vi "UHR-Fleezers Control (host) - 10.4.vi"() -> ()   [LabVIEW 2011] (continued)
            n1300 = local write "Manipulating Trap"(TRUE ("Manipulating Trap")) -> ()
            n1301 = local write "Coords"(T7 {"Horizontal"=0, "Vertical"=0} ("Coords")) -> ()
            n1302 = while {
              tunnel: w1981 -> [w1986]
              tunnel: w1979 -> [w1985]
              tunnel: w1977 -> [w1984]
              tunnel: w1976 -> [w1983]
              tunnel: w1975 -> [w1982]
              stop <- w1987 stop-if-true
              n1303 = event shown="[0] \"Pane\": Mouse Move" {
                selector: _ -> [_ _]
                dyn-events: _ -> [_ _]
                timeout: _ -> [_ _]
                tunnel: ["Force Manip Abort" w2051] -> w1987
                tunnel: w1986 -> [w1994 _]
                tunnel: w1985 -> [w1992 _]
                tunnel: w1984 -> [w1991 _]
                tunnel: w1983 -> [w1990 _]
                tunnel: w1982 -> [w1989 _]
                event Mouse Move {
                  n1304 = event-data() -> ("Time"=w1995:u32, "Coords"=w1996:T7)  [unwired: 3 out]
                  n1305 = Less?(x=w1995, y=w1994) -> (x < y?=w1993:bool)
                  n1306 = case "Makes sure old motion events prior to mouse click aren't used" shown="False" w1993 {
                    tunnel: w1996 -> [w2038 _]
                    tunnel: w1992 -> [w2039 _]
                    tunnel: w1991 -> [w2016 _]
                    tunnel: w1990 -> [w2012 _]
                    tunnel: w1989 -> [w2011 _]
                    frame False {
                      n1307 = Subtract(x=w2038, y=w2039) -> (x-y=w2037:T7)
                      "Coords" <- w2037
                      n1308 = local read "Y RF Frequency Limits (MHz)"() -> (w1997:T16)
                      n1309 = To Double Precision Float(number=w2037) -> (double precision float=w2036:cluster{"Horizontal":dbl, "Vertical":dbl})
                      n1310 = Multiply(x=cluster{"Horizontal":dbl, "Vertical":dbl} {"Horizontal"=-1.0, "Vertical"=1.0}, y="Manipulation Scaling") -> (x*y=w2032:cluster{"Horizontal":dbl, "Vertical":dbl})
                      n1311 = local read "X RF Frequency Limits (MHz)"() -> (w1998:T16)
                      n1312 = Multiply(x=w2036, y=w2032) -> (x*y=w2034:cluster{"Horizontal":dbl, "Vertical":dbl})
                      n1313 = Unbundle By Name(w2034) -> ("Horizontal"=w2029:dbl, "Vertical"=w2033:dbl)
                      n1314 = Unbundle By Name(w1997) -> ("Maximum"=w2000:dbl, "Minimum"=w1999:dbl)
                      n1315 = Boolean To (0,1)(Boolean="Manip. X?") -> (0, 1=w2027:i16)
                      n1316 = Boolean To (0,1)(Boolean="Manip. Y?") -> (0, 1=w2024:i16)
                      n1317 = local read "BD 1 Frequency 2 (MHz)"() -> (w2014:dbl)
                      n1318 = Multiply(x=w2033, y=w2024) -> (x*y=w2026:dbl)
                      n1319 = Multiply(x=w2027, y=w2029) -> (x*y=w2030:dbl)
                      n1320 = local read "BD 2 Frequency 2 (MHz)"() -> (w2013:dbl)
                      n1321 = Unbundle By Name(w1998) -> ("Maximum"=w2002:dbl, "Minimum"=w2001:dbl)
                      n1322 = Add(x=w2011, y=w2026) -> (x+y=w2004:dbl)
                      n1323 = Add(x=w2012, y=w2030) -> (x+y=w2006:dbl)
                      n1324 = In Range and Coerce(upper limit=w2002, x=w2006, lower limit=w2001) -> (coerced(x)=w2005:dbl)  [unwired: 1 out]
                      n1325 = In Range and Coerce(upper limit=w2000, x=w2004, lower limit=w1999) -> (coerced(x)=w2003:dbl)  [unwired: 1 out]
                      n1326 = Subtract(x=w2005, y=w2014) -> (x-y=w2023:dbl)
                      n1327 = Subtract(x=w2003, y=w2013) -> (x-y=w2022:dbl)
                      n1328 = Square(x=w2023) -> (x^2=w2021:dbl)
                      n1329 = Square(x=w2022) -> (x^2=w2020:dbl)
                      n1330 = Add(x=w2021, y=w2020) -> (x+y=w2019:dbl)
                      n1331 = Square Root(x=w2019) -> (sqrt(x)=w2015:dbl)
                      n1332 = In Range and Coerce(upper limit="Limit Max (MHz)", x=w2015, lower limit="Limit Min (MHz)") -> (In Range?=w2008:bool)  [unwired: 1 out]
                      n1333 = Not(x="Limits Enable") -> (.not. x?=w2007:bool)
                      n1334 = Or(x=w2008, y=w2007) -> (x .or. y?=w2009:bool)
                      n1335 = case shown="True" w2009 {
                        tunnel: w2016 -> [_ w2049]
                        tunnel: w2015 -> [_ w2040]
                        tunnel: w2005 -> [_ w2047]
                        tunnel: w2014 -> [_ w2046]
                        tunnel: w2003 -> [_ w2045]
                        tunnel: w2013 -> [_ w2044]
                        tunnel: w1998 -> [_ w2042]
                        tunnel: w1997 -> [_ w2041]
                        frame False {
                        }
                        frame True {
                          n1336 = local read "BD 1 Frequency 3 (MHz)"() -> (w2048:dbl)
                          n1337 = local read "BD 2 Frequency 3 (MHz)"() -> (w2043:dbl)
                          n1338 = local write "Trap Delta (MHz)"(w2040) -> ()
                          n1339 = call "set RF board frequency - interlace.vi"("Board 2 Frequency Limits"=w2041, "Board 1 Frequency Limits"=w2042, "FPGA VI Reference In"=w2049, "Board 2 Frequency 3 (MHz)"=w2043, "Board 1 Frequency 3 (MHz)"=w2048, "Board 2 Frequency 2 (MHz)"=w2044, "Board 2 Frequency 1 (MHz)"=w2045, "Board 1 Frequency 2 (MHz)"=w2046, "Board 1 Frequency 1  (MHz)"=w2047) -> ()  [unwired: 1 in, 2 out]
                          n1340 = local write "BD 2 Frequency 1 (MHz)"(w2045) -> ()
                          n1341 = local write "BD 1 Frequency 1 (MHz)"(w2047) -> ()
                        }
                      }
                    }
                    frame True {
                    }
                  }
                }
                event Mouse Up {
                  n1342 = event-data() -> ("Button"=w2050:u16)  [unwired: 8 out]
                  n1343 = case shown="3" w2050 {
                    tunnel: [FALSE TRUE] -> w2051
                    frame 0, Default {
                    }
                    frame 3 {
                      n1344 = local read "Trap Delta (MHz)"() -> (w2053:dbl)
                      n1345 = property on="Initial delta (MHz)" class="DigNum (strict)"("Val(Sgnl)"=w2053) -> ()  [unwired: 2 in, 2 out]
                      n1346 = local write "Manipulating Trap"(FALSE ("Manipulating Trap")) -> ()
                    }
                  }
                }
              }
            }
          }
        }
      }
      event Mouse Move {
        n1347 = event-data() -> ()  [unwired: 6 out]
      }
    }
    n1348 = local read "Stop All"() -> (w1872:bool)
    n1349 = node-c288() -> ()  [unwired: 2 out]
  }
  n1350 = timed-loop "Oscillate Trap/AOM (fishing, debugging)" {
    tunnel: w38 -> [w2057]
    tunnel: [w2056] -> w83
    timing: w78 -> [_]
    timing-out: [_] -> w77
    stop <- w2056 stop-if-true
    n1351 = node-c288() -> ()  [unwired: 2 out]
    n1352 = event shown="[0] \"Oscillate Set 1\", \"Fish for Tether\": Value Change" {
      selector: _ -> [_ _ _]
      dyn-events: _ -> [_ _ _]
      timeout: _ -> [_ _ _]
      tunnel: w2057 -> [w2064 _ _]
      tunnel: [FALSE ("Stop All") _ w2353] -> w2056
      event "Oscillate Set 1", "Fish for Tether": Value Change {
        n1353 = event-data() -> ()  [unwired: 6 out]
        n1354 = local read "Oscillate Set 1"() -> (w2063:bool)
        n1355 = Or(x=w2063, y="Fish for Tether") -> (x .or. y?=w2061:bool)
        n1356 = case shown="True" w2061 {
          tunnel: w2064 -> [_ w2067]
          tunnel: "Fish for Tether" -> [_ w2066]
          frame False {
          }
          frame True {
            n1357 = case shown="True" w2066 {
              selector: w2066 -> [w2070 w2077]
              tunnel: [w2070 w2077] -> w2065
              frame False {
              }
              frame True {
                n1358 = local write "Scan axis 2"(TRUE) -> ()
                n1359 = local write "Tether"(FALSE ("Tether")) -> ()
                n1360 = property on="Trap Delta (MHz)" class="DigNum (strict)"("Val(Sgnl)"="Furthest Delta (MHz)") -> ()  [unwired: 2 in, 2 out]
                n1361 = local read "Sample Channel\nFlow"() -> (w2074:bool)
                n1362 = Not(x=w2074) -> (.not. x?=w2072:bool)
                n1363 = And(x=w2072, y="Flow ON during \nfishing?") -> (x .and. y?=w2071:bool)
                n1364 = Wait (ms)(milliseconds to wait=u32 500) -> ()  [unwired: 1 out]
                n1365 = case shown="True" w2071 {
                  selector: w2071 -> [_ w2080]
                  frame False {
                  }
                  frame True {
                    n1366 = property on="Sample Channel\nFlow" class="Bool (strict)"("Val(Sgnl)"=w2080) -> ()  [unwired: 2 in, 2 out]
                  }
                }
              }
            }
            n1367 = node-c288() -> (w2069:T21)  [unwired: 4 out]
            n1368 = timed-loop "Oscillate AOD" {
              timing: w2069 -> [_]
              timing-out: [_] -> w2068
              tunnel: w2067 -> [w2088]
              tunnel: w2065 -> [w2081]
              i -> [w2090]
              stop <- w2087 stop-if-true
              n1369 = node-c288() -> (w2089:i64)  [unwired: 1 out]
              n1370 = flat-sequence {
                tunnel: w2090 -> [w2117]
                tunnel: w2089 -> [w2116]
                tunnel: w2088 -> [w2095]
                tunnel: w2081 -> [w2098]
                tunnel: [w2098] -> w2086
                tunnel: [w2097] -> w2085
                tunnel: [w2094] -> w2084
                tunnel: [w2091] -> w2082
                tunnel: w2086 -> [w2153]
                tunnel: w2085 -> [w2151]
                tunnel: w2084 -> [w2150]
                tunnel: [w2149] -> w2083
                tunnel: w2082 -> [w2148]
                tunnel: [w2227] -> w2087
                tunnel: w2083 -> [w2226]
                frame #0 {
                  n1371 = Divide(x=w2116, y=i64 1000) -> (x/y=w2111:dbl)
                  n1372 = Multiply(x=w2111, y=w2117) -> (x*y=w2113:dbl)
                  n1373 = local read "BD 1 Frequency 2 (MHz)"() -> (w2096:dbl)
                  n1374 = Multiply(x="Osc. freq. (Hz)", y=6.283185307179586) -> (x*y=w2114:dbl)
                  n1375 = Multiply(x=w2114, y=w2113) -> (x*y=w2093:dbl)
                  n1376 = local read "BD 1 Frequency 1 (MHz)"() -> (w2101:dbl)
                  n1377 = case shown="True" w2098 {
                    tunnel: w2093 -> [w2123 w2128]
                    tunnel: w2101 -> [_ w2139]
                    tunnel: w2096 -> [_ w2140]
                    tunnel: [w2120 w2134] -> w2099
                    tunnel: [FALSE w2131] -> w2094
                    tunnel: [0.0 w2124] -> w2091
                    frame False {
                      n1378 = Sine(x=w2123) -> (sin(x)=w2121:dbl)
                      n1379 = Multiply(x=w2121, y="Osc. amp. (MHz)") -> (x*y=w2120:dbl)
                    }
                    frame True {
                      n1380 = Cosine(x=w2128) -> (cos(x)=w2143:dbl)
                      n1381 = Subtract(x=w2140, y=w2139) -> (x-y=w2138:dbl)
                      n1382 = Decrement(x=w2143) -> (x-1=w2142:dbl)
                      n1383 = Subtract(x=w2138, y="Closest Delta (MHz)") -> (x-y=w2135:dbl)
                      n1384 = Divide(x=w2142, y=-2.0) -> (x/y=w2136:dbl)
                      n1385 = Multiply(x=w2136, y=w2135) -> (x*y=w2134:dbl)
                      n1386 = local read "Vec Mean of T1 T2"() -> (w2130:dbl[])
                      n1387 = Greater?(x=w2130, y="Stop F (pN)") -> (0:w2132:bool[])
                      n1388 = Or Array Elements(Boolean array=w2132) -> (logical OR=w2131:bool)
                      n1389 = Divide(x=w2128, y=6.283185307179586) -> (x/y=w2127:dbl)
                      n1390 = Round Toward +Infinity(x=w2127) -> (ceil(x): smallest int >= x=w2124:dbl)
                      "Attempts" <- w2124
                      n1391 = Greater?(x=w2124, y="Attempt Limit") -> (0:w2126:bool)
                      n1392 = case shown="True" w2126 {
                        frame False {
                        }
                        frame True {
                          n1393 = local write "Fish for Tether"(FALSE ("Fish for Tether")) -> ()
                          n1394 = call <vilib>:"Beep.vi"() -> ()  [unwired: 3 in, 9 out]
                          n1395 = local read "Messages"() -> (w2145:string)
                          n1396 = call "Update messages.vi"("Message to add"="Tether fishing timeout." ("Messages"), "Old message string"=w2145) -> ("New message string"=→"Messages":string)
                        }
                      }
                    }
                  }
                  n1397 = local read "BD 2 Frequency 1 (MHz)"() -> (w2100:dbl)
                  n1398 = Select(t=w2101, s="Scan axis 2", f=w2100) -> (s? t:f=w2104:dbl)
                  n1399 = Add(x=w2099, y=w2104) -> (x+y=w2097:dbl)
                  n1400 = Select(t=w2097, s="Scan axis 2", f=w2101) -> (s? t:f=w2107:dbl)
                  n1401 = Select(t=w2100, s="Scan axis 2", f=w2097) -> (s? t:f=w2106:dbl)
                  n1402 = local read "Y RF Frequency Limits (MHz)"() -> (w2102:T16)
                  n1403 = local read "X RF Frequency Limits (MHz)"() -> (w2103:T16)
                  n1404 = local read "BD 1 Frequency 3 (MHz)"() -> (w2110:dbl)
                  n1405 = local read "BD 2 Frequency 2 (MHz)"() -> (w2109:dbl)
                  n1406 = local read "BD 2 Frequency 3 (MHz)"() -> (w2108:dbl)
                  n1407 = call "set RF board frequency - interlace.vi"("Board 2 Frequency Limits"=w2102, "Board 1 Frequency Limits"=w2103, "FPGA VI Reference In"=w2095, "Board 2 Frequency 3 (MHz)"=w2108, "Board 1 Frequency 3 (MHz)"=w2110, "Board 2 Frequency 2 (MHz)"=w2109, "Board 2 Frequency 1 (MHz)"=w2106, "Board 1 Frequency 2 (MHz)"=w2096, "Board 1 Frequency 1  (MHz)"=w2107) -> ()  [unwired: 1 in, 2 out]
                }
                frame #1 {
                  n1408 = And(x=w2153, y=w2150) -> (x .and. y?=w2152:bool)
                  n1409 = case "Only if were fishing and now formed tether" shown="True" w2152 {
                    tunnel: w2151 -> [w2155 w2172]
                    tunnel: [w2154 w2171] -> w2149
                    tunnel: w2148 -> [_ w2167]
                    frame False {
                      n1410 = local read "Fish for Tether"() -> (w2154:bool)
                      n1411 = case shown="False" w2154 {
                        tunnel: w2155 -> [w2156 _]
                        frame False {
                          n1412 = property on="BD 1 Frequency 1 (MHz)" class="DigNum (strict)"("Val(Sgnl)"=w2156) -> ()  [unwired: 2 in, 2 out]
                        }
                        frame True {
                        }
                      }
                    }
                    frame True {
                      w2171 = FALSE ("Fish for Tether")
                      n1413 = call <vilib>:"Beep.vi"() -> ()  [unwired: 3 in, 9 out]
                      n1414 = Number To Decimal String(number=w2167, width (-)=i16 1) -> (decimal integer string=w2165:string)
                      n1415 = Concatenate Strings("Formed tether in ", w2165, " attempt(s)." ("string")) -> (w2162:string)
                      n1416 = local read "Messages"() -> (w2169:string)
                      n1417 = local write "Fish for Tether"(w2171) -> ()
                      n1418 = call "Update messages.vi"("Message to add"=w2162, "Old message string"=w2169) -> ("New message string"=w2168:string)
                      n1419 = local write "Messages"(w2168) -> ()
                      n1420 = Get Date/Time In Seconds() -> (seconds since 1Jan1904=→"Time tether formed":timestamp)
                      n1421 = local read "Sample Channel\nFlow"() -> (w2160:bool)
                      n1422 = local read "Flow ON during \nfishing?"() -> (w2159:bool)
                      n1423 = And(x=w2160, y=w2159) -> (x .and. y?=w2158:bool)
                      n1424 = case shown="True" w2158 {
                        tunnel: [_ w2174] -> w2157
                        frame False {
                        }
                        frame True {
                          n1425 = property on="Sample Channel\nFlow" class="Bool (strict)"("Val(Sgnl)"=FALSE ("Value (Signaling)")) -> (error out=w2174:errorcluster)  [unwired: 2 in, 1 out]
                        }
                      }
                      n1426 = case shown="\"2\", \"3\", \"4\", \"5\", \"6\"" "Then..." {
                        selector: "Then..." -> [_ w2177]
                        tunnel: w2172 -> [w2176 _]
                        tunnel: w2157 -> [_ _]
                        frame "1", Default {
                          n1427 = property on="BD 1 Frequency 1 (MHz)" class="DigNum (strict)"("Val(Sgnl)"=w2176) -> ()  [unwired: 2 in, 2 out]
                        }
                        frame "2", "3", "4", "5", "6" {
                          n1428 = flat-sequence {
                            tunnel: w2177 -> [w2179]
                            frame #0 {
                              n1429 = property on="Trap Delta (MHz)" class="DigNum (strict)"("Val(Sgnl)"="Move to Delta 1 (MHz)") -> ()  [unwired: 2 in, 2 out]
                            }
                            frame #1 {
                              n1430 = case shown="\"5\", \"6\"" w2179 {
                                selector: w2179 -> [w2182 w2192 _]
                                frame "3", "4" {
                                n1431 = flat-sequence {
                                tunnel: w2182 -> [w2183]
                                tunnel: [w2183] -> w2180
                                tunnel: [w2185] -> w2181
                                tunnel: w2180 -> [w2185]
                                tunnel: w2181 -> [w2189]
                                frame #0 {
                                n1432 = property on="Green Laser ON/Interlacing" class="Bool (strict)"("Val(Sgnl)"=TRUE ("Value (Signaling)")) -> ()  [unwired: 2 in, 2 out]
                                }
                                frame #1 {
                                n1433 = Multiply(x="Wait Before Save (s)", y=u32 1000 ("x")) -> (x*y=w2187:u32)
                                n1434 = Wait (ms)(milliseconds to wait=w2187) -> ()  [unwired: 1 out]
                                }
                                frame #2 {
                                n1435 = property on="Start Saving" class="Bool (strict)"("Value"=TRUE ("Start Saving")) -> ()  [unwired: 2 in, 2 out]
                                n1436 = case shown="\"4\"" w2189 {
                                frame Default {
                                }
                                frame "4" {
                                n1437 = property on="Fl. Triggered..." class="Bool (strict)"("Val(Sgnl)"=TRUE ("Value (Signaling)")) -> ()  [unwired: 2 in, 2 out]
                                }
                                }
                                }
                                }
                                }
                                frame "5", "6" {
                                n1438 = stacked-sequence {
                                tunnel: w2192 -> [_ _ _ _ _ _ w2204]
                                frame #0 {
                                n1439 = Replace Array Subset(array=u32[] [0] ("Index Values"), new element="Raster Set Upon Tether", index=0) -> (w2193:u32[])
                                n1440 = property on="Saved AOD Raster Scan Parameter Sets" class="Arr (strict)"("Index Values"=w2193) -> ()  [unwired: 2 in, 2 out]
                                }
                                frame #1 {
                                n1441 = Wait (ms)(milliseconds to wait=u32 500) -> ()  [unwired: 1 out]
                                }
                                frame #2 {
                                n1442 = property on="Load parameters" class="Bool (strict)"("Val(Sgnl)"=TRUE ("Value (Signaling)")) -> ()  [unwired: 2 in, 2 out]
                                n1443 = case shown="True" "Green ON During Raster" {
                                frame False {
                                }
                                frame True {
                                n1444 = property on="Green Laser ON/Interlacing" class="Bool (strict)"("Val(Sgnl)"=TRUE ("Value (Signaling)")) -> ()  [unwired: 2 in, 2 out]
                                }
                                }
                                }
                                frame #3 {
                                n1445 = Wait (ms)(milliseconds to wait=u32 500) -> ()  [unwired: 1 out]
                                }
                                frame #4 {
                                n1446 = property on="Trap Raster Scan" class="Bool (strict)"("Val(Sgnl)"=TRUE ("Value (Signaling)")) -> ()  [unwired: 2 in, 2 out]
                                }
                                frame #5 {
                                n1447 = Wait (ms)(milliseconds to wait=u32 2000) -> ()  [unwired: 1 out]
                                }
                                frame #6 {
                                n1448 = flat-sequence {
                                tunnel: w2204 -> [w2211]
                                frame #0 {
                                n1449 = while {
                                stop <- w2207 stop-if-true
                                n1450 = local read "Raster Scanning..."() -> (w2206:bool)
                                n1451 = local read "Saving..."() -> (w2209:bool)
                                n1452 = Wait (ms)(milliseconds to wait=u32 100) -> ()  [unwired: 1 out]
                                n1453 = Not(x=w2209) -> (.not. x?=w2208:bool)
                                n1454 = Not(x=w2206) -> (.not. x?=w2205:bool)
                                n1455 = And(x=w2208, y=w2205) -> (x .and. y?=w2207:bool)
                                }
                                }
                                frame #1 {
                                n1456 = local read "Tether"() -> (w2212:bool)
                                n1457 = case shown="False" w2212 {
                                tunnel: w2211 -> [_ w2214]
                                frame False {
                                n1458 = property on="Fish for Tether" class="Bool (strict)"("Val(Sgnl)"="Fish again after \nraster break?") -> ()  [unwired: 2 in, 2 out]
                                }
                                frame True {
                                n1459 = stacked-sequence {
                                tunnel: w2214 -> [_ w2216 _ _]
                                frame #0 {
                                n1460 = property on="Trap Delta (MHz)" class="DigNum (strict)"("Val(Sgnl)"="Move to Delta 2 (MHz)") -> ()  [unwired: 2 in, 2 out]
                                }
                                frame #1 {
                                n1461 = flat-sequence {
                                tunnel: w2216 -> [w2218]
                                frame #0 {
                                n1462 = Wait (ms)(milliseconds to wait=u32 500) -> ()  [unwired: 1 out]
                                }
                                frame #1 {
                                n1463 = case shown="\"6\"" w2218 {
                                frame Default {
                                }
                                frame "6" {
                                n1464 = property on="Green Laser ON/Interlacing" class="Bool (strict)"("Val(Sgnl)"=TRUE ("Green Laser ON/Interlacing")) -> ()  [unwired: 2 in, 2 out]
                                }
                                }
                                }
                                frame #2 {
                                n1465 = Wait (ms)(milliseconds to wait=u32 500) -> ()  [unwired: 1 out]
                                }
                                frame #3 {
                                n1466 = local write "Start Saving"("Save at end (5, 6)") -> ()
                                }
                                }
                                }
                                frame #2 {
                                n1467 = local read "Bead Sep. Int. Time (s)"() -> (w2224:dbl)
                                n1468 = Multiply(x=w2224, y=1000.0) -> (x*y=w2223:dbl)
                                n1469 = Wait (ms)(milliseconds to wait=w2223) -> ()  [unwired: 1 out]
                                }
                                frame #3 {
                                n1470 = property on="Rescale on Mean" class="Bool (strict)"("Val(Sgnl)"=TRUE ("Value (Signaling)")) -> ()  [unwired: 2 in, 2 out]
                                }
                                }
                                }
                                }
                                }
                                }
                                }
                                }
                                }
                                frame "2", Default {
                                }
                              }
                            }
                          }
                        }
                      }
                      "Tether" <- "Tether Alarm?"
                    }
                  }
                }
                frame #2 {
                  n1471 = local read "Oscillate Set 1"() -> (w2231:bool)
                  n1472 = local read "Stop All"() -> (w2229:bool)
                  n1473 = Or(x=w2231, y=w2226) -> (x .or. y?=w2228:bool)
                  n1474 = Not(x=w2228) -> (.not. x?=w2230:bool)
                  n1475 = Compound Arithmetic op=OR(w2229, w2230) -> (w2227:bool)
                }
              }
              n1476 = node-c288() -> ()  [unwired: 2 out]
            }
            n1477 = node-c288(w2068) -> ()  [unwired: 1 out]
          }
        }
      }
      event "Fl. Triggered...": Value Change {
        n1478 = event-data() -> ()  [unwired: 7 out]
        n1479 = case shown="True" "Fl. Triggered..." {
          frame False {
          }
          frame True {
            n1480 = node-c288() -> (w2241:T21)  [unwired: 4 out]
            n1481 = timed-loop {
              timing: w2241 -> [_]
              timing-out: [_] -> w2240
              tunnel: "Action" -> [w2245]
              shift-right: [w2242] -> _
              shift-left: u8 255 -> [w2244]
              stop <- w2246 stop-if-true
              n1482 = node-c288() -> ()  [unwired: 2 out]
              n1483 = flat-sequence {
                tunnel: w2245 -> [w2258]
                tunnel: w2244 -> [w2255]
                tunnel: [w2254] -> w2243
                tunnel: [w2344] -> w2246
                tunnel: w2243 -> [w2343]
                tunnel: [w2343] -> w2242
                frame #0 {
                  n1484 = local read "Delta Fl. 2"() -> (w2249:dbl)
                  n1485 = local read "Delta Fl. 1"() -> (w2250:dbl)
                  n1486 = Select(t=w2250, s="APD to Watch", f=w2249) -> (s? t:f=w2248:dbl)
                  n1487 = Multiply(x="Fl. Delta Thresh. (kHz)", y=1000.0) -> (x*y=w2257:dbl)
                  n1488 = Greater?(x=w2248, y=w2257) -> (0:w2252:bool)
                  n1489 = Or(x="Force Yank", y=w2252) -> (x .or. y?=w2253:bool)
                  n1490 = case shown="True" w2253 {
                    tunnel: w2258 -> [_ w2268]
                    tunnel: w2255 -> [w2260 w2264]
                    tunnel: [w2260 w2261] -> w2254
                    frame False {
                    }
                    frame True {
                      n1491 = flat-sequence {
                        tunnel: w2265 -> [w2274]
                        tunnel: [w2274] -> w2269
                        tunnel: w2268 -> [w2273]
                        tunnel: [w2273] -> w2267
                        tunnel: [w2272] -> w2266
                        tunnel: w2264 -> [w2271]
                        tunnel: [w2270] -> w2263
                        tunnel: w2269 -> [w2299]
                        tunnel: w2267 -> [w2298]
                        tunnel: w2266 -> [w2297]
                        tunnel: w2263 -> [w2296]
                        tunnel: [w2296] -> w2262
                        tunnel: w2262 -> [w2341]
                        tunnel: [w2341] -> w2261
                        frame #0 {
                          n1492 = call <vilib>:"Beep.vi"() -> ()  [unwired: 3 in, 9 out]
                          n1493 = local write "Waiting"(FALSE ("Waiting")) -> ()
                          n1494 = Increment(x=w2271) -> (x+1=w2270:u8)
                          n1495 = case shown="\"Yank\"" w2273 {
                            tunnel: w2270 -> [_ _ w2280]
                            frame "Image" {
                              n1496 = property on="Confocal Image" class="Bool (strict)"("Val(Sgnl)"=TRUE ("Value (Signaling)")) -> ()  [unwired: 2 in, 2 out]
                            }
                            frame "Alarm", Default {
                            }
                            frame "Yank" {
                              n1497 = flat-sequence {
                                tunnel: w2280 -> [w2283]
                                tunnel: [w2282] -> w2279
                                tunnel: ["N Array El"] -> w2278
                                tunnel: w2279 -> [w2293]
                                tunnel: w2278 -> [w2289]
                                frame #0 {
                                n1498 = Multiply(x="Yank Delay (s)", y=1000.0) -> (x*y=w2286:dbl)
                                n1499 = Quotient & Remainder(x=w2283, y="N Array El") -> (x-y*floor(x/y)=w2282:u8)  [unwired: 1 out]
                                n1500 = Wait (ms)(milliseconds to wait=w2286) -> ()  [unwired: 1 out]
                                }
                                frame #1 {
                                n1501 = Random Number (0-1)() -> (number: 0 to 1=w2290:dbl)
                                n1502 = Multiply(x=w2289, y=w2290) -> (x*y=w2288:dbl)
                                n1503 = Round Toward -Infinity(1:w2288) -> (0:w2287:dbl)
                                n1504 = Select(t=w2287, s="Random Choice", f=w2293) -> (s? t:f=w2291:dbl)
                                n1505 = Index Array(array="Yank to Delta Array (MHz)", index=w2291) -> (element=w2294:dbl)
                                n1506 = property on="Trap Delta (MHz)" class="DigNum (strict)"("Val(Sgnl)"=w2294) -> ()  [unwired: 2 in, 2 out]
                                }
                              }
                            }
                          }
                          n1507 = local read "Time (s)"() -> (w2272:dbl)
                          "Fl. High" <- TRUE ("Yanking")
                        }
                        frame #1 {
                          n1508 = node-c288() -> (w2301:T21)  [unwired: 4 out]
                          n1509 = timed-loop {
                            timing: w2301 -> [_]
                            timing-out: [_] -> w2300
                            tunnel: w2299 -> [w2317]
                            tunnel: w2298 -> [w2315]
                            tunnel: w2297 -> [w2314]
                            stop <- w2316 stop-if-true
                            n1510 = node-c288() -> ()  [unwired: 2 out]
                            n1511 = local read "Fl. Delta Thresh. (kHz)"() -> (w2309:dbl)
                            n1512 = local read "Fl. Triggered..."() -> (w2318:bool)
                            n1513 = local read "Delta Fl. 1"() -> (w2305:dbl)
                            n1514 = local read "Delta Fl. 2"() -> (w2303:dbl)
                            n1515 = local read "Stop All"() -> (w2312:bool)
                            n1516 = local read "APD to Watch"() -> (w2304:bool)
                            n1517 = Select(t=w2305, s=w2304, f=w2303) -> (s? t:f=w2302:dbl)
                            n1518 = Not(x=w2318) -> (.not. x?=w2313:bool)
                            n1519 = Multiply(x=w2309, y=1000.0) -> (x*y=w2308:dbl)
                            n1520 = Negate(x=w2308) -> (-x=w2307:dbl)
                            n1521 = Less?(x=w2302, y=w2307) -> (x < y?=w2311:bool)
                            n1522 = Compound Arithmetic op=OR(w2311, w2312, w2313, "Force Reset") -> (w2316:bool)
                            n1523 = case shown="True" w2316 {
                              tunnel: w2317 -> [_ w2329]
                              tunnel: w2315 -> [_ w2328]
                              tunnel: w2314 -> [_ w2326]
                              frame False {
                              }
                              frame True {
                                n1524 = case shown="\"Yank\"" w2328 {
                                tunnel: w2329 -> [_ w2330]
                                frame "Image", Default {
                                }
                                frame "Yank" {
                                n1525 = flat-sequence {
                                tunnel: [w2335] -> w2331
                                tunnel: w2330 -> [w2335]
                                tunnel: w2331 -> [w2336]
                                frame #0 {
                                n1526 = local read "Yank Delay (s)"() -> (w2334:dbl)
                                n1527 = Multiply(x=w2334, y=1000.0) -> (x*y=w2332:dbl)
                                n1528 = Wait (ms)(milliseconds to wait=w2332) -> ()  [unwired: 1 out]
                                }
                                frame #1 {
                                n1529 = property on="Trap Delta (MHz)" class="DigNum (strict)"("Val(Sgnl)"=w2336) -> ()  [unwired: 2 in, 2 out]
                                }
                                }
                                }
                                }
                                n1530 = local read "Time (s)"() -> (w2327:dbl)
                                n1531 = Subtract(x=w2327, y=w2326) -> (x-y=w2323:dbl)
                                "Duration (s)" <- w2323
                                n1532 = Number To Decimal String(number=w2323, width (-)=i16 0) -> (decimal integer string=w2321:string)
                                n1533 = Concatenate Strings(w2321, " s fluorescence event." ("string")) -> (w2319:string)
                                n1534 = local read "Messages"() -> (w2325:string)
                                n1535 = call "Update messages.vi"("Message to add"=w2319, "Old message string"=w2325) -> ("New message string"=w2324:string)
                                n1536 = call <vilib>:"Beep.vi"() -> ()  [unwired: 3 in, 9 out]
                                n1537 = local write "Messages"(w2324) -> ()
                              }
                            }
                            n1538 = node-c288() -> ()  [unwired: 2 out]
                          }
                          n1539 = node-c288(w2300) -> ()  [unwired: 1 out]
                        }
                        frame #2 {
                          n1540 = local write "Fl. High"(FALSE ("Yanking")) -> ()
                        }
                      }
                      n1541 = local read "Trap Delta (MHz)"() -> (w2265:dbl)
                    }
                  }
                }
                frame #1 {
                  n1542 = local read "Stop All"() -> (w2347:bool)
                  n1543 = local read "Fl. Triggered..."() -> (w2345:bool)
                  n1544 = Not(x=w2345) -> (.not. x?=w2346:bool)
                  n1545 = Or(x=w2346, y=w2347) -> (x .or. y?=w2344:bool)
                  n1546 = Not(x=w2344) -> (.not. x?=→"Waiting":bool)
                }
              }
              n1547 = node-c288() -> ()  [unwired: 2 out]
            }
            n1548 = node-c288(w2240) -> ()  [unwired: 1 out]
          }
        }
      }
      event "Stop All": Value Change {
        n1549 = event-data() -> ()  [unwired: 7 out]
        n1550 = local read "Stop All"() -> (w2353:bool)
      }
    }
    n1551 = node-c288() -> ()  [unwired: 2 out]
  }
  n1552 = flat-sequence "Video" {
    tunnel: [w2362] -> w68
    tunnel: w68 -> [w2403]
    frame #0 {
      n1553 = while {
        stop <- w2355 continue-if-true
        n1554 = call "Close Video Capture.vi"() -> ("error code OUT"=w2357:i32)
        n1555 = Equal?(x=w2357, y=0) -> (x = y?=w2355:bool)
      }
      n1556 = local write "Stop All"(FALSE ("Stop All")) -> ()
    }
    frame #1 {
      n1557 = call "DMR_Init.vi"() -> ()  [unwired: 3 out]
    }
    frame #2 {
      # "Setting the destination format to Mono8 makes sure that the image can be displayed in the intensity plot."
      n1558 = call "DMR_GetDevice.vi"("search string IN"="DE019116701") -> ("device handle OUT"=w2380:i32)  [unwired: 4 in, 2 out]
      n1559 = call "DMR_OpenDevice.vi"("device handle IN"=w2380) -> ("driver handle OUT"=w2363:i32)  [unwired: 4 out]
      n1560 = call "DMR_FindList.vi"("flags IN"=u32 0 ("flags"), "list name IN"="" ("String"), "list type IN"=T31."camera descriptions", "driver handle IN"=w2363) -> ("list handle OUT"=w2366:i32)  [unwired: 2 out]
      n1561 = call "DMR_FindList.vi"("flags IN"=u32 0 ("flags"), "list name IN"="Base", "list type IN"=T31."setting", "driver handle IN"=w2363) -> ("list handle OUT"=w2364:i32)  [unwired: 2 out]
      n1562 = call "OBJ_GetHandle.vi"("object name IN"="VideoStandard", "list handle IN"=w2366) -> ("object handle OUT"=w2360:i32)  [unwired: 3 out]
      n1563 = call "OBJ_GetHandle.vi"("object name IN"="PixelFormat", "list handle IN"=w2364) -> ("object handle OUT"=w2374:i32)  [unwired: 3 out]
      n1564 = call "OBJ_SetS.vi"("value index IN"=0, "value IN"="NTSC M", "object handle IN"=w2360) -> ()  [unwired: 2 out]
      n1565 = call "OBJ_SetS.vi"("value index IN"=0, "value IN"="Mono8" ("value"), "object handle IN"=w2374) -> ()  [unwired: 2 out]
      n1566 = call "OBJ_GetHandle.vi"("object name IN"="VideoChannel", "list handle IN"=w2364) -> ("object handle OUT"=w2370:i32)  [unwired: 3 out]
      n1567 = while {
        tunnel: [w2385] -> w2362
        tunnel: w2363 -> [w2382]
        stop <- w2383 continue-if-true
        n1568 = call "DMR_ImageRequestSingle.vi"("request control IN"=0, "driver handle IN"=w2382) -> ("error code OUT"=w2384:i32, "driver handle OUT"=w2385:i32)  [unwired: 2 out]
        n1569 = Equal To 0?(x=w2384) -> (x = 0?=w2383:bool)
      }
      n1570 = call "OBJ_SetI.vi"("value index IN"=0, "value IN"=3 ("Video channel"), "object handle IN"=w2370) -> ()  [unwired: 2 out]
    }
    frame #3 {
      w2391 = T17 0 items=["Grayscale (U8)", "Grayscale (I16)", "Grayscale (SGL)", "Complex (CSG)", "RGB (U32)", "HSL (U32)", "RGB (U64)"] ("Image Type")
      w2399 = T17 0 items=["Grayscale (U8)", "Grayscale (I16)", "Grayscale (SGL)", "Complex (CSG)", "RGB (U32)", "HSL (U32)", "RGB (U64)"] ("Image Type")
      n1571 = for "Create Greyscale map" {
        N: 256 -> [_]
        tunnel: [w2405] -> w2388 mode=indexing
        workers-P: _ -> [_]
        i -> [w2408]
        n1572 = To Unsigned Byte Integer(number=w2408) -> (unsigned 8bit integer=w2404:u8)
        n1573 = Join Numbers(hi=w2404, lo=w2404) -> ((hi.lo)=w2407:u16)
        n1574 = Join Numbers(hi=w2404, lo=w2404) -> ((hi.lo)=w2406:u16)
        n1575 = Join Numbers(hi=w2407, lo=w2406) -> ((hi.lo)=w2405:u32)
      }
      n1576 = call "IMAQ Create"("Image Name"="Scaled video", "Image Type"=w2391) -> ("New Image"=w2390:T2)  [unwired: 2 in, 2 out]
      n1577 = call "IMAQ Create"("Image Name"="Main video", "Image Type"=w2399) -> ("New Image"=w2400:T2)  [unwired: 2 in, 2 out]
      n1578 = node-c288(0 ("Processor")) -> (w2398:T21)  [unwired: 3 out]
      n1579 = Initialize Array(u32 0 ("Window Number (0...15)"), 480 ("dimension size"), 640 ("dimension size")) -> (w2393:u32[][])
      n1580 = timed-loop {
        tunnel: w2403 -> [w2425]
        tunnel: [w2424] -> w2402
        tunnel: w2400 -> [w2423]
        timing: w2398 -> [_]
        timing-out: [_] -> w2397
        tunnel: w2393 -> [w2412]
        tunnel: w2390 -> [w2410]
        tunnel: w2388 -> [w2409]
        stop <- w2411 stop-if-true
        # "This block performs the \nactual image capture."
        n1581 = node-c288() -> ()  [unwired: 2 out]
        n1582 = local read "Stop All"() -> (w2411:bool)
        n1583 = Reciprocal(x="Video Capture Rate (Hz)") -> (1/x=w2415:dbl)
        n1584 = Multiply(x=w2415, y=1000.0) -> (x*y=w2413:dbl)
        n1585 = call "DMR_ImageRequestWaitFor.vi"("queue number IN"=0, "timeout(ms) IN"=500, "driver handle IN"=w2425) -> ("error code OUT"=w2429:i32, "request number OUT"=w2426:i32, "driver handle OUT"=w2427:i32)
        n1586 = feedback #1(T32 refnum ("Avi Refnum")) -> (w2417:T32)
        n1587 = case shown="True" "New Video File" {
          tunnel: [T32 refnum ("Avi Refnum") w2446] -> w2419
          tunnel: [FALSE TRUE] -> w2420
          tunnel: w2417 -> [_ w2442]
          frame False {
          }
          frame True {
            n1588 = call "Create new save file.vi"("Ext"=".avi" ("string"), "Index In"="Video Index") -> ("Path Out"=w2438:path, "Index Out"=w2439:dbl)  [unwired: 1 in]
            "Path Out" <- w2438
            n1589 = Not Equal?(x=w2442, y=T32 refnum ("Avi Refnum")) -> (x != y?=w2443:bool)
            n1590 = Increment(x=w2439) -> (x+1=w2448:dbl)
            n1591 = case shown="True" w2443 {
              tunnel: w2442 -> [_ w2449]
              frame False {
              }
              frame True {
                n1592 = call "IMAQ AVI Close"("Avi Refnum"=w2449) -> ()  [unwired: 1 in, 10 out]
              }
            }
            n1593 = local write "Video Index"(w2448) -> ()
            n1594 = call "IMAQ AVI Create"("Frames Per Second"=u32 30, "AVI Path"=w2438) -> ("Avi Refnum"=w2446:T32)  [unwired: 5 in, 4 out]
          }
        }
        n1595 = Equal To 0?(x=w2429) -> (x = 0?=w2428:bool)
        n1596 = Select(t=w2419, s=w2420, f=w2417) -> (s? t:f=w2418:T32)
        n1597 = feedback-in #1(w2418) -> ()
        n1598 = case shown="True" w2428 {
          tunnel: w2427 -> [w2450 w2475]
          tunnel: w2426 -> [_ w2474]
          tunnel: [w2450 w2471] -> w2424
          tunnel: w2423 -> [_ w2455]
          tunnel: w2412 -> [_ w2459]
          tunnel: w2418 -> [_ w2457]
          tunnel: w2410 -> [_ w2452]
          tunnel: w2409 -> [_ w2451]
          frame False {
          }
          frame True {
            w2465 = u32 0 ("X-offset IN")
            n1599 = call "DMR_GetImageRequestBufferData.vi"("driver handle IN"=w2475, "request number IN"=w2474) -> ("width OUT"=w2464:i32, "height OUT"=w2463:i32, "driver handle OUT"=w2470:i32, "request number OUT"=w2469:i32, "bytes per pixel OUT"=w2466:i32)  [unwired: 13 out]
            n1600 = call "DMR_GetImageRequestBufferImageData.vi"("driver handle IN"=w2470, "request number IN"=w2469, "bytes per pixel IN"=w2466, "X-offset IN"=w2465, "Y-offset IN"=w2465, "height IN"=w2463, "width IN"=w2464) -> ("driver handle OUT"=w2468:u32, "request number OUT"=w2467:u32, "image OUT"=w2460:u32[][])  [unwired: 10 out]
            n1601 = call "DMR_ImageRequestUnlock.vi"("request number IN"=w2467, "driver handle IN"=w2468) -> ("driver handle OUT"=w2473:i32)  [unwired: 1 in, 2 out]
            n1602 = case shown="True" "Averaging" {
              tunnel: w2460 -> [w2511 w2516]
              tunnel: [w2511 w2515] -> w2456
              tunnel: w2459 -> [_ w2513]
              frame False {
              }
              frame True {
                (unwired) 1
                w2521 = 1
                n1603 = feedback #2(w2513) -> (w2512:u32[][])
                n1604 = Add(x=w2516, y=w2512) -> (x+y=w2517:u32[][])
                n1605 = Select(t=w2513, s="Reset Averaging", f=w2517) -> (s? t:f=w2519:u32[][])
                n1606 = feedback-in #2(w2519) -> ()
                n1607 = feedback #3(w2521) -> (w2514:i32)
                n1608 = Divide(x=w2517, y=w2514) -> (x/y=w2518:dbl[][])
                n1609 = Increment(x=w2514) -> (x+1=w2522:i32)
                n1610 = To Unsigned Long Integer(number=w2518) -> (unsigned 32bit integer=w2515:u32[][])
                n1611 = Select(t=w2521, s="Reset Averaging", f=w2522) -> (s? t:f=w2520:i32)
                n1612 = feedback-in #3(w2520) -> ()
              }
            }
            n1613 = call "DMR_ImageRequestSingle.vi"("request control IN"=0, "driver handle IN"=w2473) -> ("driver handle OUT"=w2471:i32)  [unwired: 3 out]
            n1614 = disable-structure shown="Disabled" {
              disable-tunnel: w2456 -> [w2488 _]
              disable-tunnel: w2452 -> [w2487 _]
              frame Disabled {
                n1615 = To Double Precision Float(number=w2488) -> (double precision float=w2486:dbl[][])
                n1616 = In Range and Coerce(upper limit="Intensity Upper", x=w2486, lower limit="Intensity Lower") -> (coerced(x)=w2485:dbl[][])  [unwired: 1 out]
                n1617 = Subtract(x="Intensity Upper", y="Intensity Lower") -> (x-y=w2482:dbl)
                n1618 = Subtract(x=w2485, y="Intensity Lower") -> (x-y=w2483:dbl[][])
                n1619 = Divide(x=w2483, y=w2482) -> (x/y=w2484:dbl[][])
                n1620 = Multiply(x=255.0, y=w2484) -> (x*y=w2480:dbl[][])
                n1621 = To Unsigned Byte Integer(number=w2480) -> (unsigned 8bit integer=w2489:u8[][])
                n1622 = call "IMAQ ArrayToImage"("Image Pixels (U8)"=w2489, "Image"=w2487) -> ("Image Out"=w2476:T2)  [unwired: 4 in, 5 out]
                n1623 = First Call?() -> (First Call?: T/F=w2477:bool)
                n1624 = case shown="True" w2477 {
                  tunnel: w2476 -> [w2490 w2501]
                  frame False {
                    n1625 = flat-sequence {
                      tunnel: w2490 -> [w2496]
                      frame #0 {
                        w2493 = FALSE ("Get/Set Status? (Set)")
                        w2492 = 0 ("Window Number (0...15)")
                        n1626 = call "IMAQ WindSize"("Get/Set Status? (Set)"=w2493, "Window Number"=w2492) -> ("Width & Height out"=→"Window Size":cluster{"Width":i32, "Height":i32})  [unwired: 4 in, 2 out]
                        n1627 = call "IMAQ WindMove"("Window Number (0...15)"=w2492, "Get/Set Status? (Set)"=w2493) -> ("Coordinates (screen)"=→"Window Position":cluster{"X Position":i32, "Y Position":i32})  [unwired: 3 in, 1 out]
                        n1628 = call "IMAQ WindDraw"("Resize to Image Size? (Y)"=FALSE, "Window Number (0...15)"=w2492, "Image"=w2496) -> ()  [unwired: 7 in, 2 out]
                      }
                      frame #1 {
                        n1629 = call "IMAQ WindZoom 2"("Center Point"="Center Point", "Zoom to Fit? (False)"=FALSE, "Zoom Factor"="Zoom Factor") -> ()  [unwired: 5 in, 4 out]
                      }
                    }
                  }
                  frame True {
                    n1630 = flat-sequence {
                      tunnel: w2501 -> [w2504]
                      tunnel: [w2502] -> w2500
                      tunnel: w2500 -> [w2506]
                      frame #0 {
                        w2503 = TRUE ("Resize to Image Size? (Y)")
                        w2502 = 0 ("Window Number (0...15)")
                        n1631 = call "IMAQ WindNonTearing"("Window Number"=w2502, "NonTearing? (True)"=w2503) -> ()  [unwired: 8 in, 2 out]
                        n1632 = call "IMAQ WindDraw"("Resize to Image Size? (Y)"=w2503, "Window Number (0...15)"=w2502, "Image"=w2504) -> ()  [unwired: 7 in, 2 out]
                      }
                      frame #1 {
                        n1633 = call "IMAQ WindSize"("Scrollbars? (N)"=FALSE, "Width & Height"="Initial Window Size", "Window Number"=w2506) -> ()  [unwired: 3 in, 3 out]
                        n1634 = call "IMAQ WindMove"("Window Number (0...15)"=w2506, "Coordinates (screen)"="Initial Window Position") -> ()  [unwired: 3 in, 2 out]
                      }
                    }
                  }
                }
              }
              frame Enabled {
              }
            }
            n1635 = To Unsigned Byte Integer(number=w2456) -> (unsigned 8bit integer=w2454:u8[][])
            n1636 = call "IMAQ ArrayToImage"("Image Pixels (U8)"=w2454, "Image"=w2455) -> ("Image Out"=w2453:T2)  [unwired: 4 in, 5 out]
            "Primary Video Display" <- w2453
            n1637 = case shown="True" "Save Video" {
              tunnel: w2457 -> [_ w2510]
              tunnel: w2453 -> [_ w2509]
              frame False {
              }
              frame True {
                n1638 = call "IMAQ AVI Write Frame"("Image"=w2509, "Avi Refnum"=w2510) -> ()  [unwired: 2 in, 8 out]
              }
            }
            n1639 = case shown="True" "Save Image" {
              tunnel: w2454 -> [_ w2525]
              tunnel: w2451 -> [_ w2524]
              frame False {
              }
              frame True {
                n1640 = call <vilib>:"Flatten Pixmap.vi"("colors"=w2524, "8-bit pixmap"=w2525) -> ("image data"=w2531:T33)  [unwired: 4 in, 5 out]
                n1641 = call "Create new save file.vi"("Insert"="video_frame_" ("string"), "Ext"=".bmp" ("string"), "Index In"="Image Index") -> ("Path Out"=w2527:path, "Index Out"=w2532:dbl)
                n1642 = Increment(x=w2532) -> (x+1=w2526:dbl)
                n1643 = local write "Image Index"(w2526) -> ()
                n1644 = call <vilib>:"Write BMP File.vi"("image data"=w2531, "path to BMP file"=w2527) -> ()  [unwired: 1 in, 9 out]
              }
            }
          }
        }
        n1645 = node-c288(w2413) -> ()  [unwired: 1 out]
      }
      n1646 = node-c288(w2397) -> ()  [unwired: 1 out]
      n1647 = call "DMR_CloseDevice.vi"("driver handle IN"=w2402) -> ()  [unwired: 1 in, 4 out]
    }
    frame #4 {
      n1648 = call "DMR_Close.vi"() -> ()  [unwired: 1 out]
    }
  }
  n1649 = node-c288(i64 1 ("Period"), 1 ("Processor")) -> (w163:T21)  [unwired: 2 out]
  n1650 = timed-loop "Acquire Data" {
    tunnel: w38 -> [w2828]
    tunnel: w37 -> [w2827]
    tunnel: [w2857] -> w258
    tunnel: [w2852] -> w256
    timing: w163 -> [_]
    timing-out: [_] -> w162
    tunnel: w57 -> [w2662]
    stop <- "Stop All" stop-if-true
    w2577 = "Initialize"
    w2647 = "NI_ChannelName" ("name")
    n1651 = node-c288() -> ()  [unwired: 2 out]
    n1652 = First Call?() -> (First Call?: T/F=w2612:bool)
    n1653 = Or(x="Reset", y=w2612) -> (x .or. y?=w2613:bool)
    n1654 = case "Reset data stream" shown="True" w2613 {
      tunnel: w2828 -> [w3799 w3807]
      tunnel: w2827 -> [w3798 w3806]
      tunnel: [w3799 w3801] -> w2823
      tunnel: [w3798 w3800] -> w2822
      frame False {
      }
      frame True {
        w3804 = TRUE ("AI to FIFO")
        n1655 = local write "Overflow (data lost)"(FALSE ("Overflow (data lost)")) -> ()
        n1656 = call "reset FPGA DMA.vi"("error in"=w3806, "FPGA VI Reference In"=w3807) -> ("error out"=w3802:errorcluster, "FPGA VI Reference Out"=w3803:T19)
        n1657 = xnode "Read/Write Control"("FPGA VI Reference In"=w3803, "error in"=w3802, "AI to FIFO"=w3804, "APD to FIFO"=w3804) -> ("FPGA VI Reference Out"=w3801:T19, "error out"=w3800:errorcluster)
      }
    }
    n1658 = Or(x="Start AOD Scan", y="Trap Raster Scan") -> (x .or. y?=w2773:bool)
    n1659 = case "Start AOM raster scan" shown="True" w2773 {
      tunnel: w2823 -> [w3649 w3659]
      tunnel: w2822 -> [w3648 w3658]
      tunnel: [w3649 w3652] -> w2821
      tunnel: [w3648 w3651] -> w2820
      frame False {
      }
      frame True {
        n1660 = case shown="True" "Restart DMA? (AOD)" {
          tunnel: [w3697 w3699] -> w3653
          tunnel: [w3696 w3698] -> w3654
          tunnel: w3659 -> [w3697 w3701]
          tunnel: w3658 -> [w3696 w3700]
          frame False {
          }
          frame True {
            n1661 = local write "Overflow (data lost)"(FALSE ("Overflow (data lost)")) -> ()
            n1662 = call "reset FPGA DMA.vi"("error in"=w3700, "FPGA VI Reference In"=w3701) -> ("error out"=w3698:errorcluster, "FPGA VI Reference Out"=w3699:T19)
          }
        }
        n1663 = local write "Trap Raster Scan"(FALSE ("Trap Raster Scan")) -> ()
        n1664 = case shown="True" "Move MCL Also?" {
          tunnel: w3654 -> [w3662 w3691]
          tunnel: w3653 -> [w3663 w3692]
          tunnel: [w3661 w3695] -> w3652
          tunnel: [w3660 w3694] -> w3651
          frame False {
            w3664 = TRUE ("AI to FIFO")
            n1665 = xnode "Read/Write Control"("FPGA VI Reference In"=w3663, "error in"=w3662, "AI to FIFO"=w3664, "APD to FIFO"=w3664, "Start scan"=w3664) -> ("FPGA VI Reference Out"=w3661:T19, "error out"=w3660:errorcluster)
          }
          frame True {
            w3688 = FALSE ("1D or 2D Scan?")
            w3693 = TRUE ("AI to FIFO")
            # "Count for MCL loop"
            # "N total cycles"
            # "N steps"
            # "V_int"
            n1666 = local read "Scan Range (nm)"() -> (w3670:dbl)
            n1667 = local read "Number of F/B Scans (AOD)"() -> (w3687:u16)
